vi "读取测试开始时间.vi"(8 "错误输入（无错误）":errorcluster, 11 "VISA资源名称":refnum<visa-resource-name>) -> (0 "错误输出":errorcluster, 2 "时间标识":timestamp, 3 "VISA资源名称输出":refnum<visa-resource-name>)   [LabVIEW 2021]
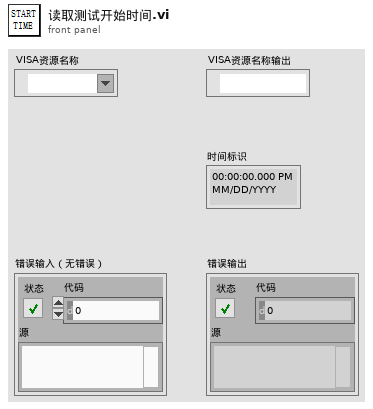
[diagram p1: front panel]
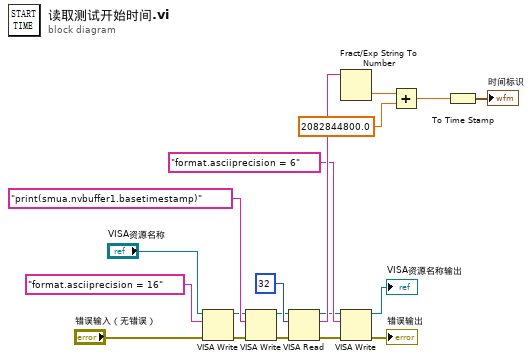
[diagram p0: block diagram]
diagram:
  n1 = VISA Write(VISA resource name="VISA资源名称", write buffer="format.asciiprecision = 16" ("格式字符串"), error in (no error)="错误输入（无错误）") -> (VISA resource name out=w2:refnum<visa-resource-name>, error out=w1:errorcluster)  [unwired: 1 out]
  n2 = VISA Write(VISA resource name=w2, write buffer="print(smua.nvbuffer1.basetimestamp)" ("格式字符串"), error in (no error)=w1) -> (VISA resource name out=w11:refnum<visa-resource-name>, error out=w10:errorcluster)  [unwired: 1 out]
  n3 = VISA Read(VISA resource name=w11, byte count=u32 32 ("字节总数"), error in (no error)=w10) -> (VISA resource name out=w9:refnum<visa-resource-name>, read buffer=w17:string, error out=w8:errorcluster)  [unwired: 1 out]
  n4 = Fract/Exp String To Number(string=w17) -> (number=w15:dbl)  [unwired: 3 in, 1 out]
  n5 = VISA Write(VISA resource name=w9, write buffer="format.asciiprecision = 6" ("格式字符串"), error in (no error)=w8) -> (VISA resource name out=→"VISA资源名称输出":refnum<visa-resource-name>, error out=→"错误输出":errorcluster)  [unwired: 1 out]
  n6 = Add(x=w15, y=2082844800.0 ("x-y")) -> (x+y=w14:dbl)
  n7 = To Time Stamp(1:w14) -> (0:→"时间标识":timestamp)
